vi "Create PID.vi"(9 "D":dbl, 10 "I":dbl, 11 "P":dbl) -> (3 "PIDClass.lvclass":refnum<class "PIDClass.lvclass">)   [LabVIEW 2012, in "PIDClass.lvclass"]
uses:
  PIDClass.lvclass
  PIDClass.lvclass/PIDClass.ctl
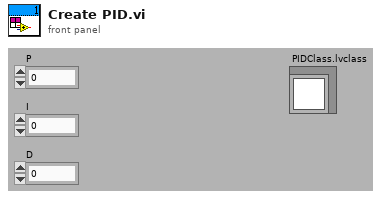
[diagram p1: front panel]
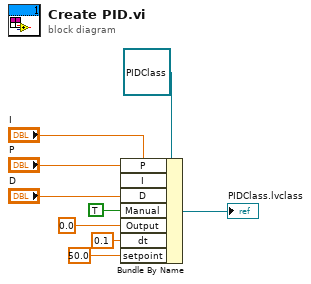
[diagram p0: block diagram]
diagram:
  n1 = Bundle By Name(cluster=refnum<class "PIDClass.lvclass"> refnum ("PIDClass.lvclass"), "P"="P", "I"="I", "D"="D", "Manual"=TRUE, "Output"=0.0, "dt"=0.1, "setpoint"=50.0) -> (→"PIDClass.lvclass":refnum<class "PIDClass.lvclass">)
